vi "SRTS_Burst_Save.vi"(7 "XLS ref.":refnum<vi>, 8 "error in":errorcluster, 10 "Burst_Result":T1, 11 "XLS in":refnum<class "XLS.lvclass">) -> (0 "error out":errorcluster, 2 "Progress":i32, 3 "XLS out":refnum<class "XLS.lvclass">)   [LabVIEW 2017, in "Report_lib.lvlib" / "XLS.lvclass"]
uses:
  XLS.lvclass
  TypeDefs/Burst_Result.ctl
  XLS.lvclass/XLS.ctl
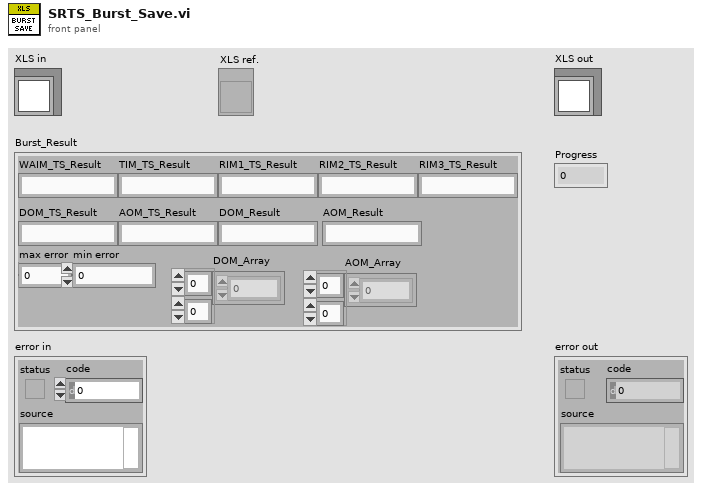
[diagram p1: front panel]
types:
  T1 = typedef "Burst_Result.ctl" = cluster{"WAIM_TS_Result":string, "DOM_TS_Result":string, "AOM_TS_Result":string, "TIM_TS_Result":string, "RIM2_TS_Result":string, "RIM1_TS_Result":string, "RIM3_TS_Result":string, "DOM_Result":string, "AOM_Result":string, "max error":dbl, "min error":dbl, "DOM_Array":dbl[][], "AOM_Array":dbl[][]}
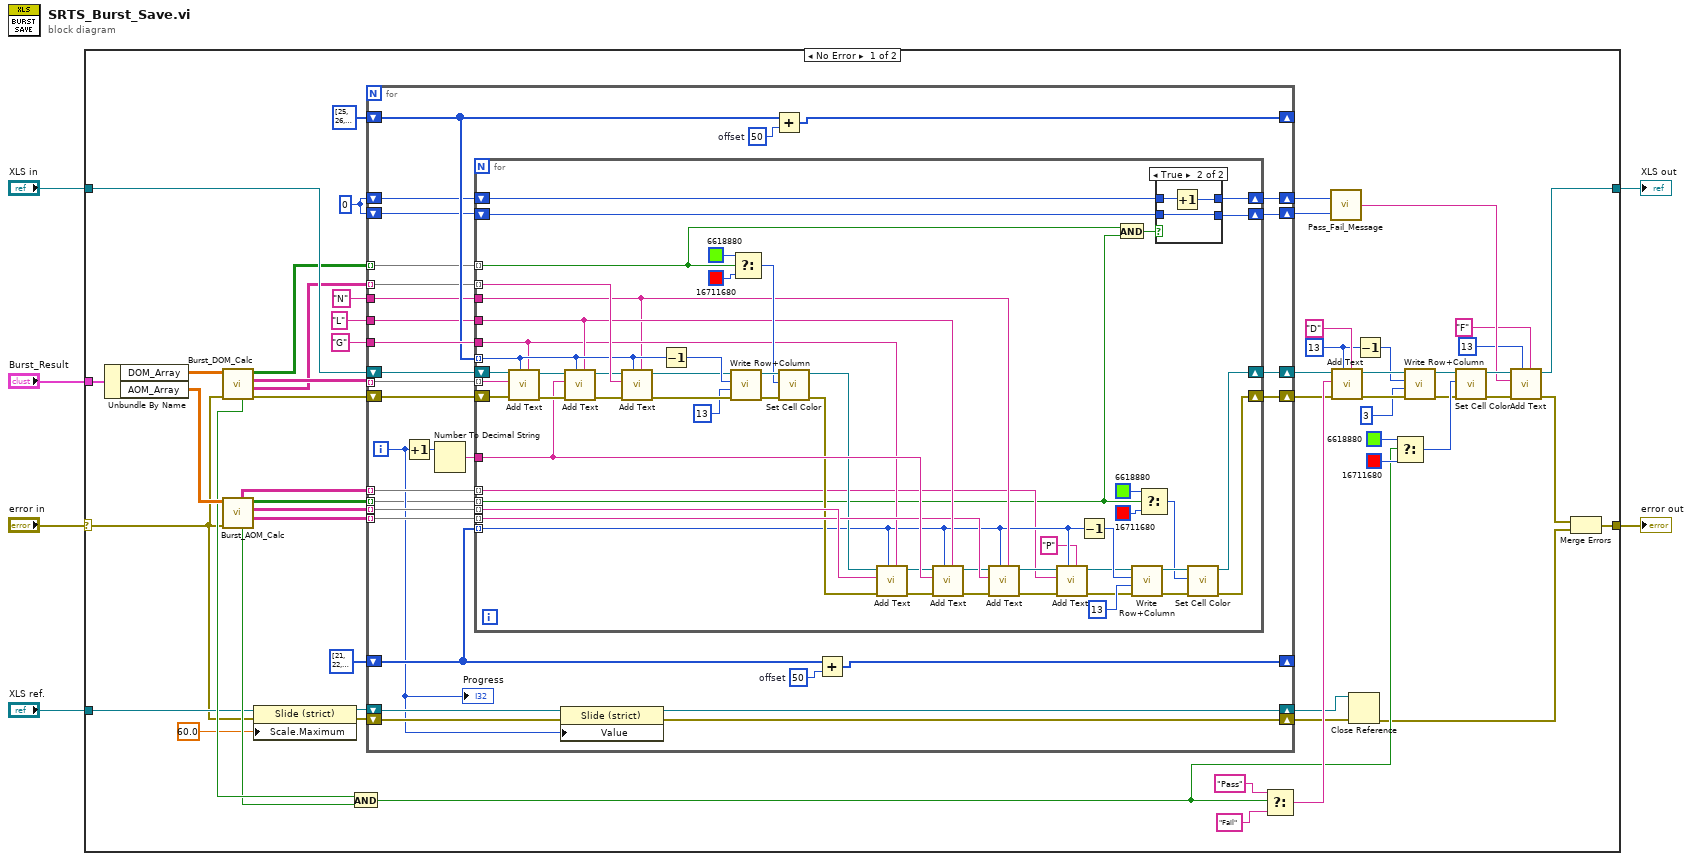
[diagram p0: block diagram]
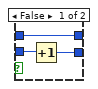
[diagram p2: hidden frame]
diagram:
  n1 = case shown="No Error" "error in" {
    selector: "error in" -> [w20 w153]
    tunnel: [w22 w153] -> w5
    tunnel: [w11 w152] -> w3
    tunnel: "XLS in" -> [w57 w152]
    tunnel: "Burst_Result" -> [w61 _]
    tunnel: "XLS ref." -> [w21 _]
    frame No Error {
      w16 = 0
      w36 = 13 ("Index")
      n2 = Unbundle By Name(w61) -> ("DOM_Array"=w60:dbl[][], "AOM_Array"=w59:dbl[][])
      n3 = call "Burst_DOM_Calc.vi"("error in"=w20, "DOM"=w60) -> ("error out"=w58:errorcluster, "DOM_Result_Str"=w48:string[][], "DOM_Values"=w50:string[][], "DOM_Result_Bool"=w49:bool[][], "DOM_Total"=w28:bool)  [unwired: 5 in]
      n4 = call "Burst_AOM_Calc.vi"("error in"=w20, "AOM"=w59) -> ("AOM_Result_Str"=w46:string[][], "AOM_Values"=w47:string[][], "AOM_Result_Bool"=w51:bool[][], "AOM_Total"=w27:bool, "Errors%"=w45:string[][])  [unwired: 4 in, 1 out]
      n5 = property class="Slide (strict)"(reference=w21, error in=w20, "Scale.Maximum"=60.0 ("Scale.Range:Maximum")) -> (reference out=w18:refnum<vi>, error out=w19:errorcluster)
      n6 = And(x=w28, y=w27) -> (x .and. y?=w26:bool)
      n7 = for {
        tunnel: "G" -> [w90]
        tunnel: w50 -> [w89] mode=indexing
        shift-right: [w85] -> _
        shift-left: i32[] [25, 26, 27, 28, 33, 34, 35, 36, 41, 42, 43, 44, 49, 50, 51, 52, 57, 58, 59, 60, 65, 66, 67, 68] ("DOM_indexies") -> [w87]
        shift-right: [w82] -> _
        shift-left: i32[] [21, 22, 23, 24, 29, 30, 31, 32, 37, 38, 39, 40, 45, 46, 47, 48, 53, 54, 55, 56, 61, 62, 63, 64] ("AOM_indexies") -> [w84]
        tunnel: w47 -> [w88] mode=indexing
        shift-right: [w81] -> w29
        shift-left: w57 -> [w91]
        shift-right: [w80] -> w30
        shift-left: w58 -> [w92]
        tunnel: "L" -> [w78]
        tunnel: "N" -> [w77]
        tunnel: w48 -> [w75] mode=indexing
        tunnel: w46 -> [w76] mode=indexing
        tunnel: w49 -> [w66] mode=indexing
        tunnel: w51 -> [w67] mode=indexing
        tunnel: w45 -> [w73] mode=indexing
        shift-right: [w70] -> w24
        shift-left: w18 -> [w72]
        shift-right: [w69] -> w25
        shift-left: w19 -> [w71]
        shift-right: [w63] -> w15
        shift-left: w16 -> [w65]
        shift-right: [w62] -> w14
        shift-left: w16 -> [w64]
        i -> [w68]
        w83 = 50  # offset
        w86 = 50  # offset
        n8 = Increment(x=w68) -> (x+1=w74:i32)
        n9 = Number To Decimal String(number=w74) -> (decimal integer string=w79:string)  [unwired: 1 in]
        n10 = for {
          shift-right: [w108] -> w81
          shift-left: w91 -> [w144]
          shift-right: [w107] -> w80
          shift-left: w92 -> [w145]
          tunnel: w87 -> [w136] mode=indexing
          tunnel: w89 -> [w143] mode=indexing
          tunnel: w90 -> [w123]
          tunnel: w84 -> [w102] mode=indexing
          tunnel: w88 -> [w132] mode=indexing
          tunnel: w79 -> [w128]
          tunnel: w78 -> [w127]
          tunnel: w77 -> [w118]
          tunnel: w76 -> [w126] mode=indexing
          tunnel: w75 -> [w142] mode=indexing
          tunnel: w66 -> [w95] mode=indexing
          tunnel: w67 -> [w94] mode=indexing
          tunnel: w73 -> [w100] mode=indexing
          shift-right: [w96] -> w63
          shift-left: w65 -> [w99]
          shift-right: [w97] -> w62
          shift-left: w64 -> [w98]
          n11 = call "Add Text.vi"("Adr"=w123, "Index"=w136, "error in"=w145, "text"=w143, "XLS in"=w144) -> ("error out"=w131:errorcluster, "XLS out"=w130:refnum<class "XLS.lvclass">)  [unwired: 5 in]
          n12 = call "Add Text.vi"("Adr"=w127, "Index"=w136, "error in"=w131, "text"=w128, "XLS in"=w130) -> ("error out"=w125:errorcluster, "XLS out"=w124:refnum<class "XLS.lvclass">)  [unwired: 5 in]
          n13 = call "Add Text.vi"("Adr"=w118, "Index"=w136, "error in"=w125, "text"=w142, "XLS in"=w124) -> ("error out"=w116:errorcluster, "XLS out"=w117:refnum<class "XLS.lvclass">)  [unwired: 5 in]
          n14 = Decrement(x=w136) -> (x-1=w135:i32)
          n15 = call "Write Row+Column.vi"("error in"=w116, "column"=13, "row"=w135, "XLS in"=w117) -> ("error out"=w141:errorcluster, "XLS out"=w140:refnum<class "XLS.lvclass">)  [unwired: 6 in]
          n16 = Select(t=u32 6618880, s=w95, f=u32 16711680) -> (s? t:f=w137:u32)
          n17 = call "Set Cell Color.vi"("error in"=w141, "color"=w137, "XLS in"=w140) -> ("error out"=w109:errorcluster, "XLS out"=w110:refnum<class "XLS.lvclass">)  [unwired: 7 in]
          n18 = call "Add Text.vi"("Adr"=w123, "Index"=w102, "error in"=w109, "text"=w132, "XLS in"=w110) -> ("error out"=w121:errorcluster, "XLS out"=w122:refnum<class "XLS.lvclass">)  [unwired: 5 in]
          n19 = call "Add Text.vi"("Adr"=w127, "Index"=w102, "error in"=w121, "text"=w128, "XLS in"=w122) -> ("error out"=w119:errorcluster, "XLS out"=w120:refnum<class "XLS.lvclass">)  [unwired: 5 in]
          n20 = call "Add Text.vi"("Adr"=w118, "Index"=w102, "error in"=w119, "text"=w126, "XLS in"=w120) -> ("error out"=w105:errorcluster, "XLS out"=w106:refnum<class "XLS.lvclass">)  [unwired: 5 in]
          n21 = call "Add Text.vi"("Adr"="P", "Index"=w102, "error in"=w105, "text"=w100, "XLS in"=w106) -> ("error out"=w104:errorcluster, "XLS out"=w103:refnum<class "XLS.lvclass">)  [unwired: 5 in]
          n22 = Decrement(x=w102) -> (x-1=w129:i32)
          n23 = And(x=w95, y=w94) -> (x .and. y?=w93:bool)
          n24 = call "Write Row+Column.vi"("error in"=w104, "column"=13, "row"=w129, "XLS in"=w103) -> ("error out"=w113:errorcluster, "XLS out"=w114:refnum<class "XLS.lvclass">)  [unwired: 6 in]
          n25 = Select(t=u32 6618880, s=w94, f=u32 16711680) -> (s? t:f=w112:u32)
          n26 = case shown="True" w93 {
            tunnel: w99 -> [w146 w150]
            tunnel: w98 -> [w148 w151]
            tunnel: [w147 w151] -> w97
            tunnel: [w146 w149] -> w96
            frame False {
              n27 = Increment(x=w148) -> (x+1=w147:i32)
            }
            frame True {
              n28 = Increment(x=w150) -> (x+1=w149:i32)
            }
          }
          n29 = call "Set Cell Color.vi"("error in"=w113, "color"=w112, "XLS in"=w114) -> ("error out"=w107:errorcluster, "XLS out"=w108:refnum<class "XLS.lvclass">)  [unwired: 7 in]
        }
        n30 = property class="Slide (strict)"(reference=w72, error in=w71, "Value"=w68) -> (reference out=w70:refnum<vi>, error out=w69:errorcluster)
        n31 = Add(x=w87, y=w86) -> (x+y=w85:i32[])
        n32 = Add(x=w84, y=w83) -> (x+y=w82:i32[])
        "Progress" <- w68
      }
      n33 = Select(t="Pass" ("Adr"), s=w26, f="Fail" ("Adr")) -> (s? t:f=w44:string)
      n34 = call "Pass_Fail_Message.vi"("Failed"=w14, "Passed"=w15) -> ("Result Message"=w9:string)
      n35 = call "Add Text.vi"("Adr"="D", "Index"=w36, "error in"=w30, "text"=w44, "XLS in"=w29) -> ("error out"=w43:errorcluster, "XLS out"=w42:refnum<class "XLS.lvclass">)  [unwired: 5 in]
      n36 = Close Reference(reference=w24, error in (no error)=w25) -> (error out=w23:errorcluster)
      n37 = Decrement(x=w36) -> (x-1=w38:i32)
      n38 = Select(t=u32 6618880, s=w26, f=u32 16711680) -> (s? t:f=w41:u32)
      n39 = call "Write Row+Column.vi"("error in"=w43, "column"=3, "row"=w38, "XLS in"=w42) -> ("error out"=w40:errorcluster, "XLS out"=w39:refnum<class "XLS.lvclass">)  [unwired: 6 in]
      n40 = call "Set Cell Color.vi"("error in"=w40, "color"=w41, "XLS in"=w39) -> ("error out"=w13:errorcluster, "XLS out"=w12:refnum<class "XLS.lvclass">)  [unwired: 7 in]
      n41 = call "Add Text.vi"("Adr"="F", "Index"=13, "error in"=w13, "text"=w9, "XLS in"=w12) -> ("error out"=w10:errorcluster, "XLS out"=w11:refnum<class "XLS.lvclass">)  [unwired: 5 in]
      n42 = Merge Errors(w10, w23) -> (w22:errorcluster)
    }
    frame Error {
    }
  }
  "error out" <- w5
  "XLS out" <- w3
